vi "Connect Channels.vi"   [LabVIEW 2016, in "SLSC Switch.lvlib" / "SLSC Switch.lvclass"]
uses:
  SLSC Switch.lvclass
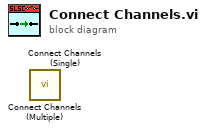
[diagram p0: block diagram]
diagram:
  n1 = call "Connect Channels (Multiple).vi"() -> ()  [unwired: 10 in, 2 out]
  n2 = call "Connect Channels (Single).vi"() -> ()  [unwired: 10 in, 2 out]
